vi "Receive Panel Close Msg.vi"(8 "error in (no error)":errorcluster, 10 "PanelCloseMsg":refnum<class "PanelCloseMsg.lvclass">, 11 "IController In":refnum<class "IController.lvclass">) -> (0 "error out":errorcluster, 3 "IController Out":refnum<class "IController.lvclass">)   [LabVIEW 2015, in "IController.lvlib" / "IController.lvclass"]
uses:
  IController.lvclass
  AutoRegistration/ActorAutoRegistration Messages/PanelCloseMsg/PanelCloseMsg.lvclass
  <vilib>/ActorFramework/Actor/Actor.lvclass/Actor.ctl
  <vilib>/ActorFramework/Message Enqueuer/Message Enqueuer.lvclass/Message Enqueuer.ctl
  <vilib>/ActorFramework/Message Enqueuer/Init from Existing Queue.vi
  <vilib>/ActorFramework/Message Enqueuer/Enqueue.vi
  <vilib>/ActorFramework/Message Priority Queue/Priority Enqueue.vi
  <vilib>/ActorFramework/Message Enqueuer/Message Enqueuer.lvclass
  <vilib>/ActorFramework/Stop Msg/Stop Msg.lvclass
  <vilib>/ActorFramework/Actor/Actor.lvclass
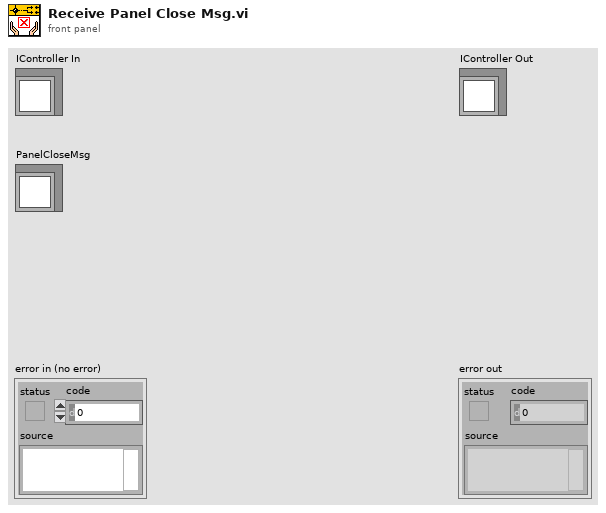
[diagram p1: front panel]
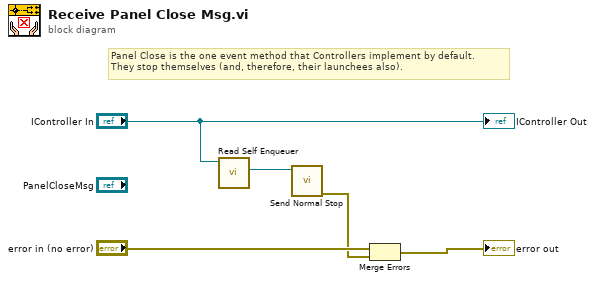
[diagram p0: block diagram]
diagram:
  # "Panel Close is the one event method that Controllers implement by default.\nThey stop themselves (and, therefore, their launchees also)."
  n1 = call <vilib>:"Read Self Enqueuer.vi"("Actor"="IController In") -> ("Self Enqueuer"=w3:refnum<class "Message Enqueuer.lvclass">)  [unwired: 10 in]
  n2 = call <vilib>:"Send Normal Stop.vi"("Message Enqueuer"=w3) -> ("error out"=w1:errorcluster)  [unwired: 10 in]
  n3 = Merge Errors("error in (no error)", w1) -> (→"error out":errorcluster)
  "IController Out" <- "IController In"
